vi "Apply Config.vi"(8 "Error In":errorcluster, 11 "object in":refnum<class "IConfigure.lvclass">) -> (0 "Error Out":errorcluster, 3 "object out":refnum<class "IConfigure.lvclass">)   [LabVIEW 2023, in "HAL.lvlib" / "PXIe-5172.lvlib" / "IConfigure.lvclass"]
uses:
  IConfigure.lvclass
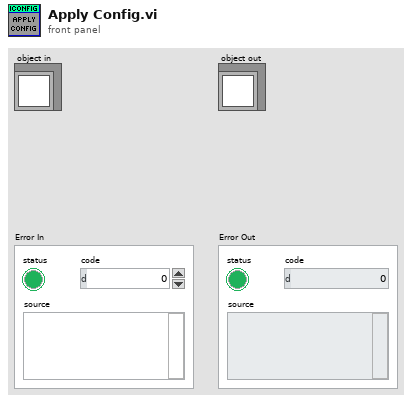
[diagram p1: front panel]
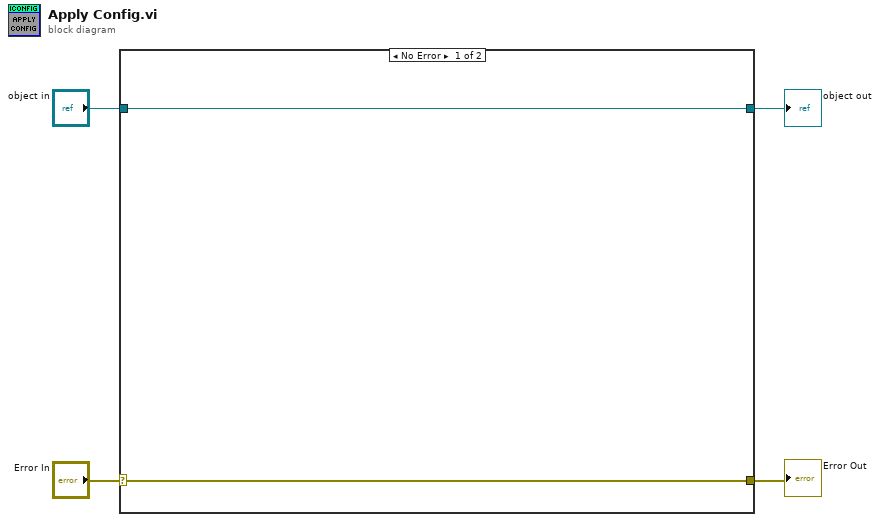
[diagram p0: block diagram]
diagram:
  n1 = case shown="No Error" "Error In" {
    selector: "Error In" -> [w6 w8]
    tunnel: [w6 w8] -> w3
    tunnel: [w5 w7] -> w1
    tunnel: "object in" -> [w5 w7]
    frame No Error {
    }
    frame Error {
    }
  }
  "Error Out" <- w3
  "object out" <- w1
